vi "G#Object_Create.vi"(0 "reference in":refnum<class "MyClass3.lvclass">, 3 "control values":variant[](array[variant]), 5 "error in (no error)":errorcluster) -> (14 "reference out":refnum<class "MyClass3.lvclass">, 19 "error out":errorcluster)   [LabVIEW 2017, in "MyClass3.lvclass"]
doc: "The G#Object default constructor."
uses:
  MyClass3.lvclass
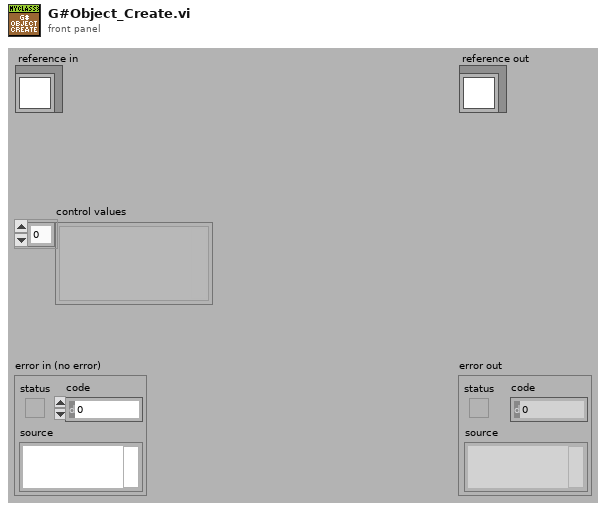
[diagram p1: front panel]
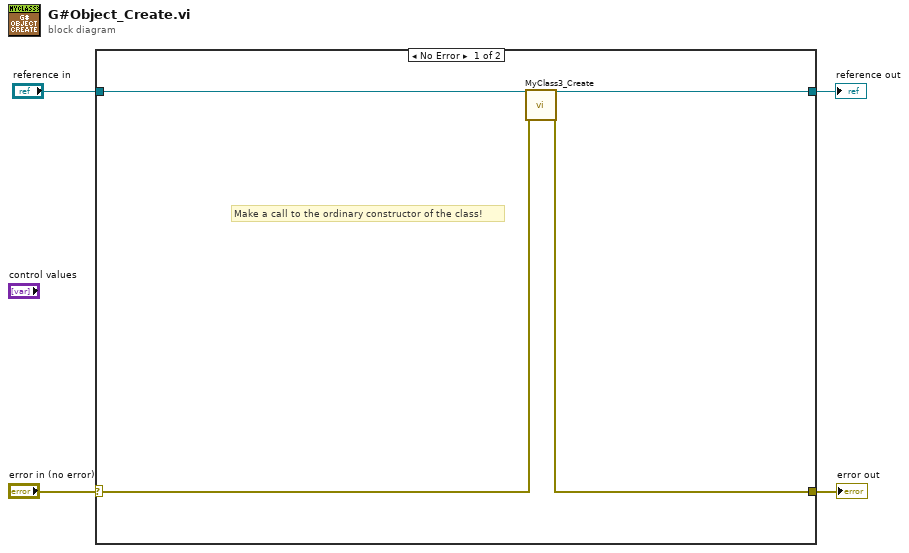
[diagram p0: block diagram]
diagram:
  n1 = case shown="No Error" "error in (no error)" {
    selector: "error in (no error)" -> [w6 w10]
    tunnel: [w5 w10] -> w3
    tunnel: [w7 w9] -> w1
    tunnel: "reference in" -> [w8 w9]
    frame No Error {
      # "Make a call to the ordinary constructor of the class!"
      n2 = call "MyClass3_Create.vi"("reference in"=w8, "error in (no error)"=w6) -> ("reference out"=w7:refnum<class "MyClass3.lvclass">, "error out"=w5:errorcluster)  [unwired: 16 in]
    }
    frame Error {
    }
  }
  "error out" <- w3
  "reference out" <- w1
